vi "Add Tag.vi"(8 "error in (no error)":errorcluster, 10 "Tag in":refnum<class "Tag.lvclass">) -> (0 "error out":errorcluster, 2 "Tag Reference out":refnum<data-value>)   [LabVIEW 2018, in "Tag Engine.lvlib" / "Tag Core.lvclass"]
uses:
  Tag Core.lvclass
  Tag/Tag.lvclass
  Tag Core.lvclass/Tag Core.ctl
  Tag/Tag.lvclass/Tag.ctl
  Tag/Read Name.vi
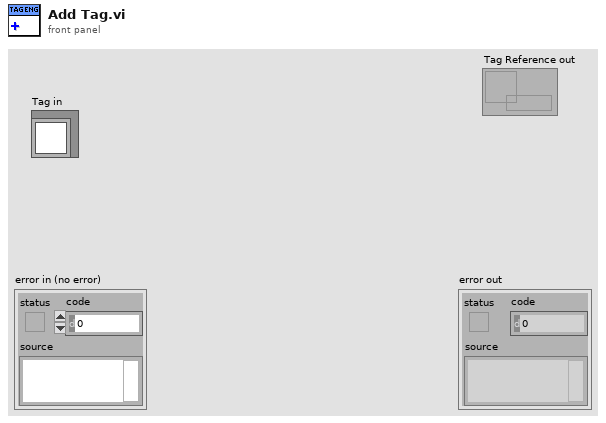
[diagram p1: front panel]
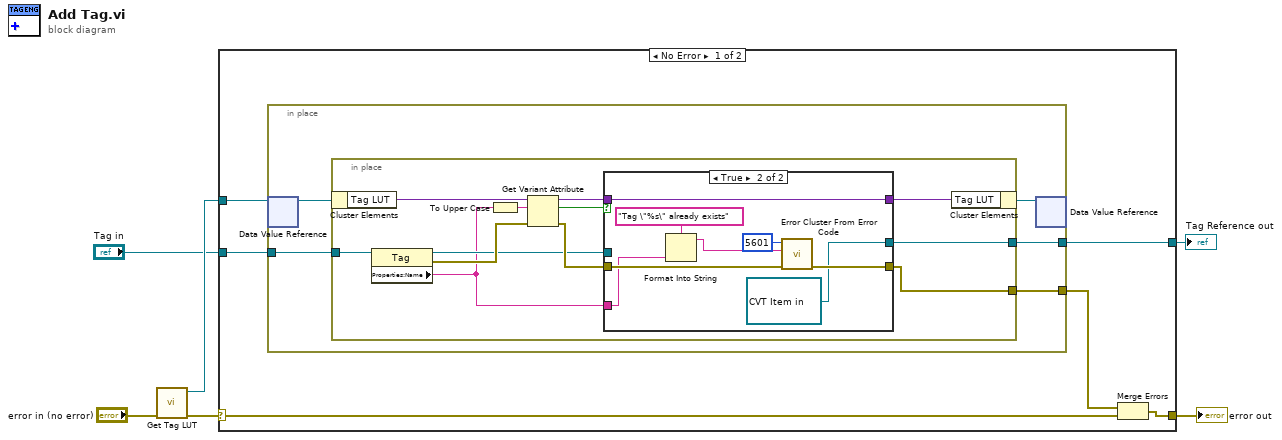
[diagram p0: block diagram]
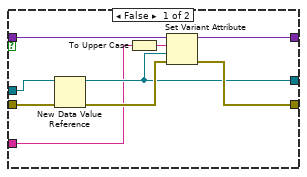
[diagram p2: hidden frame]
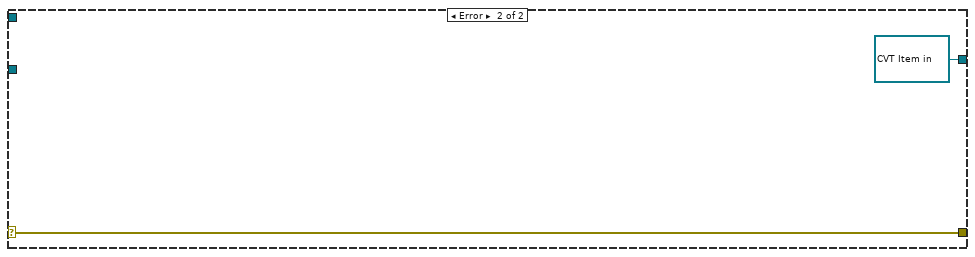
[diagram p3: hidden frame]
diagram:
  n1 = call "Get Tag LUT.vi"("error in (no error)"="error in (no error)") -> ("error out"=w4:errorcluster, "Tag LUT Out"=w3:refnum<data-value>)  [unwired: 9 in]
  n2 = case shown="No Error" w4 {
    selector: w4 -> [w11 w48]
    tunnel: [w10 w48] -> w6
    tunnel: w3 -> [w12 _]
    tunnel: "Tag in" -> [w8 _]
    tunnel: [w7 refnum<data-value> refnum ("data value reference")] -> w1
    frame No Error {
      n3 = in-place {
        in-place-border: [w15] -> w9
        in-place-border: w8 -> [w14]
        in-place-border: [w13] -> w7
        n4 = in-place-dvr #1(w12) -> (w17:refnum<class "Tag Core.lvclass">)  [unwired: 1 out]
        n5 = in-place {
          in-place-border: [w25] -> w15
          in-place-border: w14 -> [w23]
          in-place-border: [w20] -> w13
          n6 = in-place-cluster #2(w17) -> ("Tag LUT"=w28:variant)
          n7 = property class="Tag"(reference=w23) -> (reference out=w21:refnum<class "Tag.lvclass">, error out=w22:errorcluster, "Properties:Name"=w19:string)  [unwired: 1 in]
          n8 = To Upper Case(1:w19) -> (0:w18:string)
          n9 = Get Variant Attribute(Variant=w28, name=w18, error in=w22) -> (duplicate Variant=w27:variant, found=w24:bool, error out=w26:errorcluster)  [unwired: 1 in, 1 out]
          n10 = case shown="True" w24 {
            tunnel: [w38 w46] -> w29
            tunnel: w19 -> [w31 w41]
            tunnel: w21 -> [w34 _]
            tunnel: w27 -> [w37 w46]
            tunnel: w26 -> [w35 w45]
            tunnel: [w36 w44] -> w25
            tunnel: [w32 refnum<data-value> refnum ("data value reference")] -> w20
            frame False {
              n11 = New Data Value Reference(data value=w34, error in=w35) -> (data value reference=w32:refnum<data-value>, error out=w33:errorcluster)
              n12 = To Upper Case(1:w31) -> (0:w30:string)
              n13 = Set Variant Attribute(Variant=w37, name=w30, value=w32, error in=w33) -> (Variant out=w38:variant, error out=w36:errorcluster)  [unwired: 1 out]
            }
            frame True {
              n14 = Format Into String(format string="Tag \"%s\" already exists" ("error message (\"\")"), w41) -> (resulting string=w40:string)  [unwired: 2 in, 1 out]
              n15 = call <vilib>:"Error Cluster From Error Code.vi"("error in (no error)"=w45, "error message (\"\")"=w40, "error code (0)"=5601) -> ("error out"=w44:errorcluster)  [unwired: 6 in]
            }
          }
          n16 = in-place-cluster #2("Tag LUT"=w29) -> (w16:refnum<class "Tag Core.lvclass">)
        }
        n17 = in-place-dvr #1(w16) -> ()  [unwired: 2 out]
      }
      n18 = Merge Errors(w9, w11) -> (w10:errorcluster)
    }
    frame Error {
    }
  }
  "error out" <- w6
  "Tag Reference out" <- w1
